vi "Systemlink Facade.vi"(0 "Data In":T1, 2 "Display State In":T3, 3 "Container State":T4) -> (6 "Data Out":T1, 7 "Display State Out":T3, 8 "Action":T2)   [LabVIEW 2016, in "Systemlink Tag.xctl"]
uses:
  Systemlink Tag.xctl
  <vilib>/_xctls/Action.ctl
  <vilib>/_xctls/XControlSupport.lvlib
  Systemlink Data.ctl
  <vilib>/_xctls/Container State.ctl
  Systemlink State.ctl
panel:
  in  "Refresh Button":bool
  in  "Login":bool
  in  "Configure":bool
  in  "Tag":T1
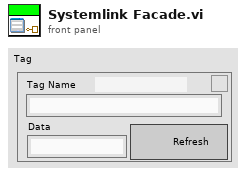
[diagram p1: front panel]
types:
  T1 = typedef "Systemlink Tag.xctl/Systemlink Data.ctl" = cluster{"Tag Name":string, "Type":string, "Data":string}
  T2 = typedef "XControlSupport.lvlib/Action.ctl" = cluster{"Data Changed?":bool, "State Changed?":bool, "Action Name":string}
  T3 = typedef "Systemlink Tag.xctl/Systemlink State.ctl" = cluster{"Numeric":dbl}
  T4 = typedef "XControlSupport.lvlib/Container State.ctl" = cluster{"Indicator?":bool, "Run Mode?":bool, " Refnum":refnum<vi>}
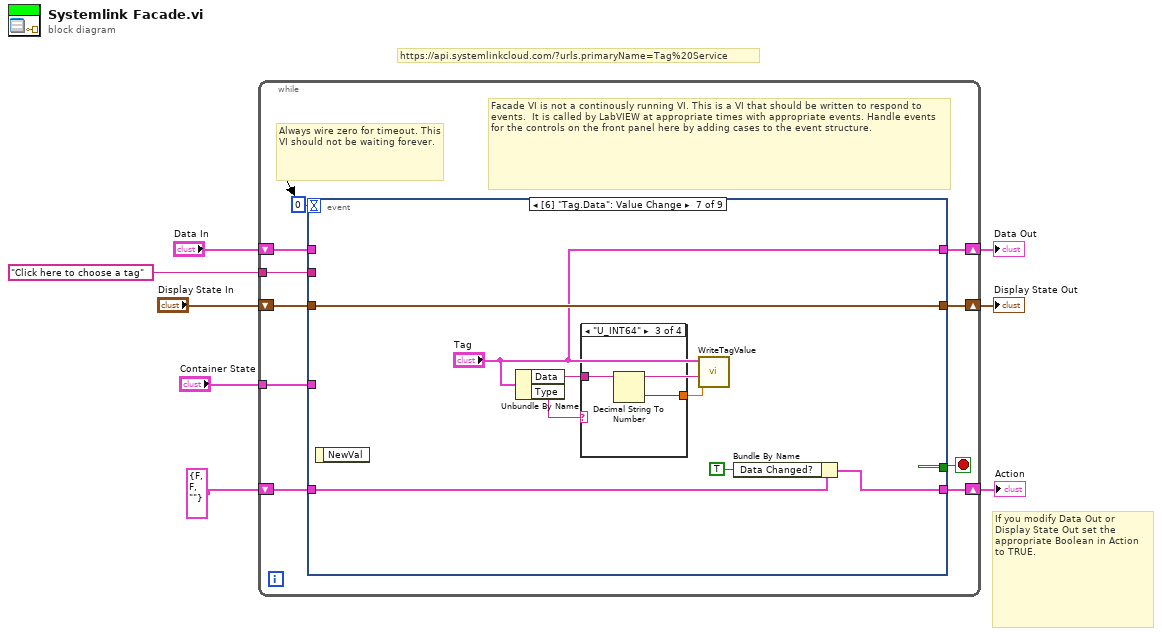
[diagram p0: block diagram]
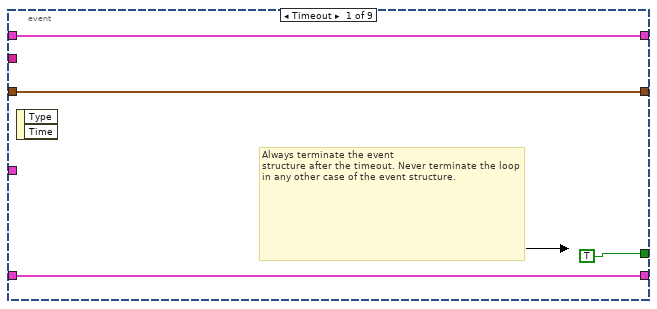
[diagram p2: hidden frame]
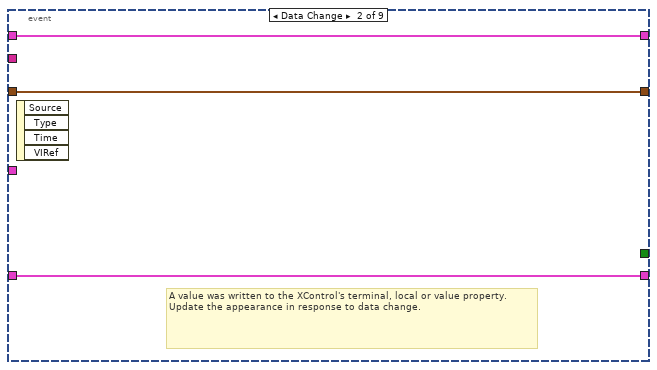
[diagram p3: hidden frame]
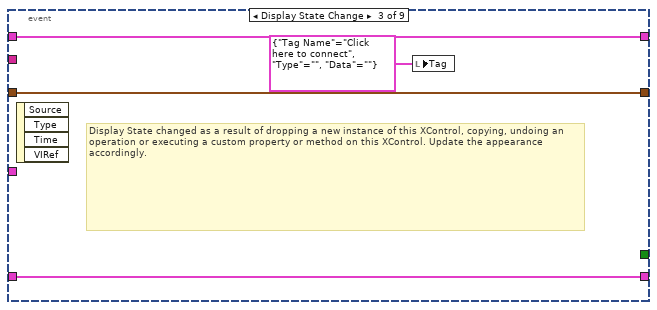
[diagram p4: hidden frame]
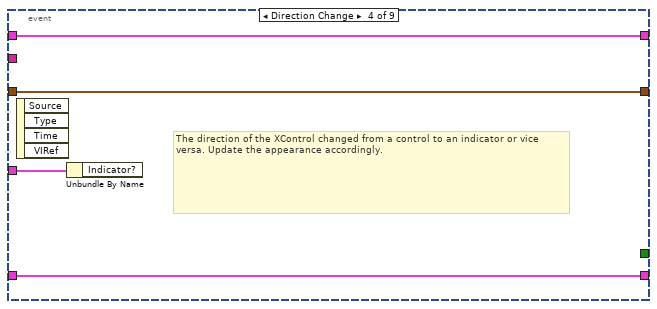
[diagram p5: hidden frame]
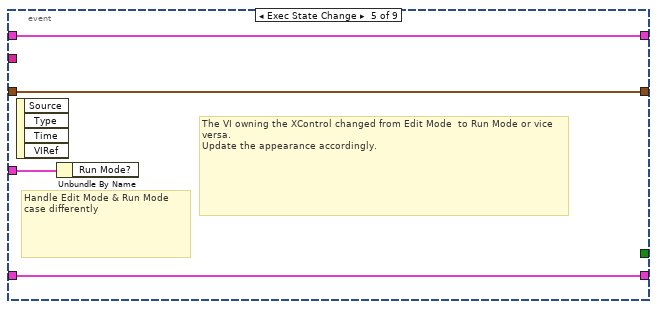
[diagram p6: hidden frame]
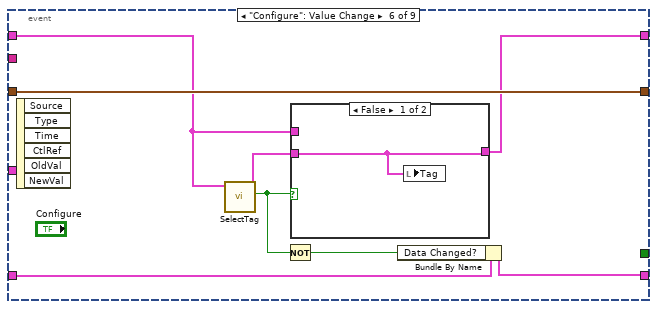
[diagram p7: hidden frame]
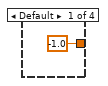
[diagram p9: hidden frame]
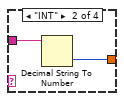
[diagram p10: hidden frame]
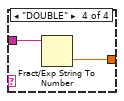
[diagram p11: hidden frame]
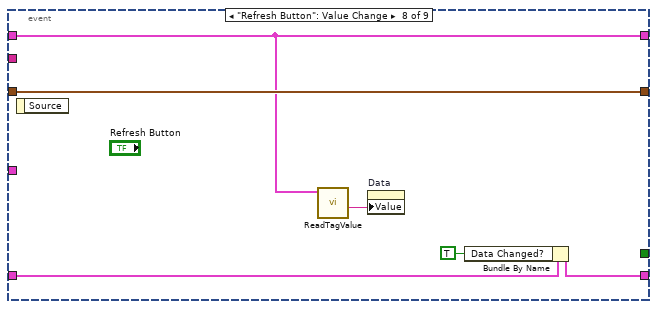
[diagram p12: hidden frame]
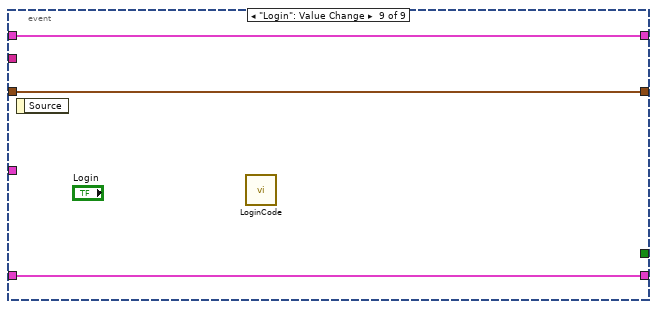
[diagram p13: hidden frame]
diagram:
  # "https://api.systemlinkcloud.com/?urls.primaryName=Tag%20Service"
  # "If you modify Data Out or\nDisplay State Out set the\nappropriate Boolean in Action\nto TRUE."
  n1 = while {
    shift-right: [w17] -> w6
    shift-left: "Display State In" -> [w18]
    tunnel: "Container State" -> [w14]
    shift-right: [w12] -> w8
    shift-left: "Data In" -> [w13]
    shift-right: [w10] -> w4
    shift-left: T2 {"Data Changed?"=FALSE, "State Changed?"=FALSE, "Action Name"=""} ("Action") -> [w11]
    tunnel: "Click here to choose a tag" -> [w9]
    stop <- w16 stop-if-true
    # "Facade VI is not a continously running VI. This is a VI that should be written to respond to events.  It is called by LabVIEW at appropriate times with appropriate events. Handle events for the controls on the front panel here by adding cases to the event structure."
    # "Always wire zero for timeout. This\nVI should not be waiting forever."
    n2 = event shown="[6] \"Tag.Data\": Value Change" {
      selector: _ -> [_ _ _ _ _ _ _ _ _]
      dyn-events: _ -> [_ _ _ _ _ _ _ _ _]
      timeout: 0 -> [_ _ _ _ _ _ _ _ _]
      tunnel: w18 -> [w20 w25 w29 w32 w36 w45 w55 w68 w71]
      tunnel: [w20 w25 w29 w32 w36 w45 w55 w68 w71] -> w17
      tunnel: [TRUE _ _ _ _ _ _ _ _] -> w16
      tunnel: w14 -> [_ _ _ w33 w37 _ _ _ _]
      tunnel: w13 -> [w19 w23 w27 w31 w35 w38 _ w67 w70]
      tunnel: [w19 w23 w27 w31 w35 w44 "Tag" w67 w70] -> w12
      tunnel: [w21 w24 w28 w30 w34 w42 w53 w64 w69] -> w10
      tunnel: w11 -> [w21 w24 w28 w30 w34 w43 w54 w66 w69]
      tunnel: w9 -> [_ _ _ _ _ _ _ _ _]
      event Timeout {
        # "Always terminate the event\nstructure after the timeout. Never terminate the loop in any other case of the event structure."
        n3 = event-data() -> ()  [unwired: 1 in, 2 out]
      }
      event Data Change {
        # "A value was written to the XControl's terminal, local or value property.\nUpdate the appearance in response to data change."
        n4 = event-data() -> ()  [unwired: 1 in, 4 out]
      }
      event Display State Change {
        # "Display State changed as a result of dropping a new instance of this XControl, copying, undoing an operation or executing a custom property or method on this XControl. Update the appearance accordingly."
        n5 = event-data() -> ()  [unwired: 1 in, 4 out]
        n6 = local write "Tag"(T1 {"Tag Name"="Click here to connect", "Type"="", "Data"=""} ("Tag")) -> ()
      }
      event Direction Change {
        # "The direction of the XControl changed from a control to an indicator or vice versa. Update the appearance accordingly."
        n7 = event-data() -> ()  [unwired: 1 in, 4 out]
        n8 = Unbundle By Name(w33) -> ()  [unwired: 1 out]
      }
      event Exec State Change {
        # "The VI owning the XControl changed from Edit Mode  to Run Mode or vice versa.\nUpdate the appearance accordingly."
        # "Handle Edit Mode & Run Mode\ncase differently"
        n9 = event-data() -> ()  [unwired: 1 in, 4 out]
        n10 = Unbundle By Name(w37) -> ()  [unwired: 1 out]
      }
      event "Configure": Value Change {
        n11 = event-data() -> ()  [unwired: 1 in, 6 out]
        n12 = call "SelectTag.vi"("Tag in"=w38) -> ("Canceled?"=w40:bool, "Tag out"=w39:T1)  [unwired: 9 in]
        n13 = Not(x=w40) -> (.not. x?=w41:bool)
        n14 = case shown="False" w40 {
          tunnel: w39 -> [w46 _]
          tunnel: [w46 w47] -> w44
          tunnel: w38 -> [_ w47]
          frame False {
            n15 = local write "Tag"(w46) -> ()
          }
          frame True {
          }
        }
        n16 = Bundle By Name(cluster=w43, "Data Changed?"=w41) -> (w42:T2)
      }
      event Value Change {
        n17 = event-data() -> ()  [unwired: 1 in, 1 out]
        n18 = Unbundle By Name("Tag") -> ("Data"=w49:string, "Type"=w50:string)
        n19 = case shown="\"U_INT64\"" w50 {
          tunnel: w49 -> [_ w58 w60 w62]
          tunnel: [-1.0 w57 w59 w61] -> w48
          frame Default {
          }
          frame "INT" {
            n20 = Decimal String To Number(string=w58) -> (number=w57:i32)  [unwired: 2 in, 1 out]
          }
          frame "U_INT64" {
            n21 = Decimal String To Number(string=w60) -> (number=w59:i32)  [unwired: 2 in, 1 out]
          }
          frame "DOUBLE" {
            n22 = Fract/Exp String To Number(string=w62) -> (number=w61:dbl)  [unwired: 3 in, 1 out]
          }
        }
        n23 = call "WriteTagValue.vi"("Number to Write"=w48, "Value"=w49, "Tag In"="Tag") -> ()  [unwired: 9 in]
        n24 = Bundle By Name(cluster=w54, "Data Changed?"=TRUE) -> (w53:T2)
      }
      event "Refresh Button": Value Change {
        n25 = event-data() -> ()  [unwired: 1 in, 1 out]
        n26 = call "ReadTagValue.vi"("Tag"=w67) -> ("Value Read"=w63:string)  [unwired: 9 in, 1 out]
        n27 = property on="Data" class="Str"("Value"=w63) -> ()  [unwired: 2 in, 2 out]
        n28 = Bundle By Name(cluster=w66, "Data Changed?"=TRUE) -> (w64:T2)
      }
      event "Login": Value Change {
        n29 = event-data() -> ()  [unwired: 1 in, 1 out]
        n30 = call "LoginCode.vi"() -> ()  [unwired: 10 in, 2 out]
      }
    }
  }
  "Display State Out" <- w6
  "Data Out" <- w8
  "Action" <- w4
